vi "Choreo_TrajectoryDifferential_Flipped.vi"(11 "ChoreoTrajectoryDifferential":T1) -> (3 "FlippedTrajectorySwerve":T1)   [LabVIEW 2019, in "ChoreoLib.lvlib"]
doc: "Returns this trajectory, mirrored across the field midline.\n\nInputs:\n -- ChoreoTrajectoryDifferential - cluster - data cluster for this trajectory \n\nOutputs: \n -- FlippedTrajectoryDifferential- cluster - this trajectory, mirrored across the field midline."
uses:
  ChoreoLib.lvlib
  TypeDef/ChoreoTrajectoryDifferential.ctl
  TypeDef/ChoreoDifferentialSample.ctl
  TypeDef/ChoreoEventMarker.ctl
  Choreo_Util_AllianceFlipGetFlipper.vi
  Choreo_Util_AllianceFlipX.vi
  Choreo_Util_AllianceFlipY.vi
  Choreo_Util_AllianceFlipHeading.vi
  Choreo_DifferentialSample_New.vi
  Choreo_Choreo_Globals.vi
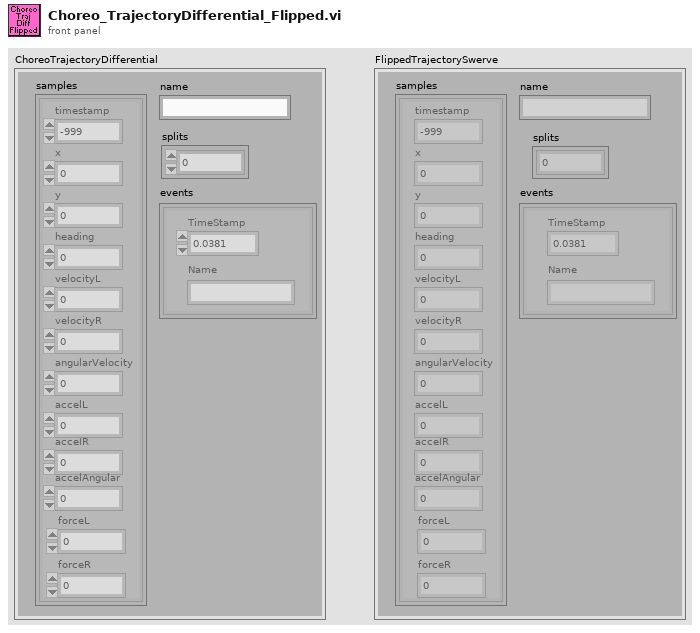
[diagram p1: front panel]
types:
  T1 = typedef "ChoreoLib.lvlib/ChoreoTrajectoryDifferential.ctl" = cluster{"name":string, "samples":T2[], "splits":i32[], "events":T3[]}
  T2 = typedef "ChoreoLib.lvlib/ChoreoDifferentialSample.ctl" = cluster{"timestamp":dbl, "x":dbl, "y":dbl, "heading":dbl, "velocityL":dbl, "velocityR":dbl, "angularVelocity":dbl, "accelL":dbl, "accelR":dbl, "accelAngular":dbl, "forceL":dbl, "forceR":dbl}
  T3 = typedef "ChoreoLib.lvlib/ChoreoEventMarker.ctl" = cluster{"TimeStamp":dbl, "Name":string}
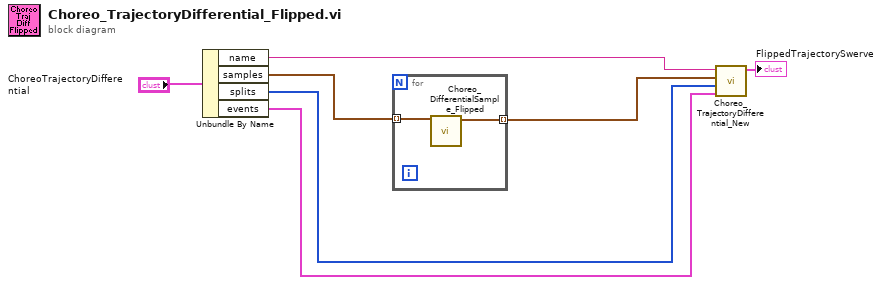
[diagram p0: block diagram]
diagram:
  n1 = Unbundle By Name("ChoreoTrajectoryDifferential") -> ("name"=w6:string, "samples"=w3:T2[], "splits"=w5:i32[], "events"=w4:T3[])
  n2 = for {
    tunnel: w3 -> [w9] mode=indexing
    tunnel: [w8] -> w2 mode=indexing
    n3 = call "Choreo_DifferentialSample_Flipped.vi"("ChoreoDifferentialSample"=w9) -> ("FlippedDifferentialSample"=w8:T2)  [unwired: 10 in]
  }
  n4 = call "Choreo_TrajectoryDifferential_New.vi"("events"=w4, "splits"=w5, "samples"=w2, "name"=w6) -> ("ChoreoTrajectoryDifferential"=→"FlippedTrajectorySwerve":T1)  [unwired: 7 in]
